vi "Apply Tombstone.vi"(5 "Time of Death (ToD)":timestamp, 7 "Grave Digger":string, 8 "Error In":errorcluster, 11 "Grave In":refnum<vi>) -> (0 "Error Out":errorcluster, 3 "Grave Out":refnum<vi>)   [LabVIEW 2017, in "Toolkit VIs.lvlib"]
doc: "Adds a tomestome to the grave. The grave is a Diagram Disable structure and the tomestone is its label as a bookmark with a \"RIP\" tag to indicate its a tomestone, the died date in YYYYMMDD format, and the name of the grave digger (programmer). \n\nBy default today's date is used as the died date and the application/system user name is used for the grave digger."
uses:
  Toolkit VIs.lvlib
  Public/Typedefs/Bookmark Tags.ctl
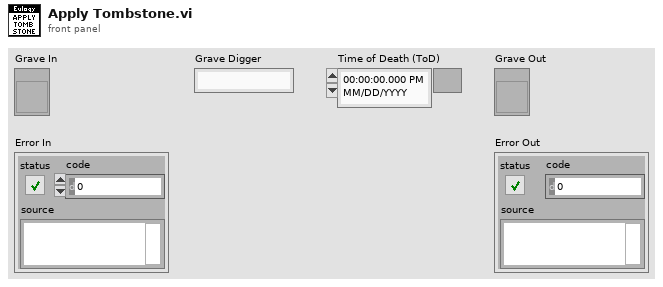
[diagram p1: front panel]
types:
  T1 = typedef "Toolkit VIs.lvlib/Bookmark Tags.ctl" = enum16{"RIP", "Zombie"}
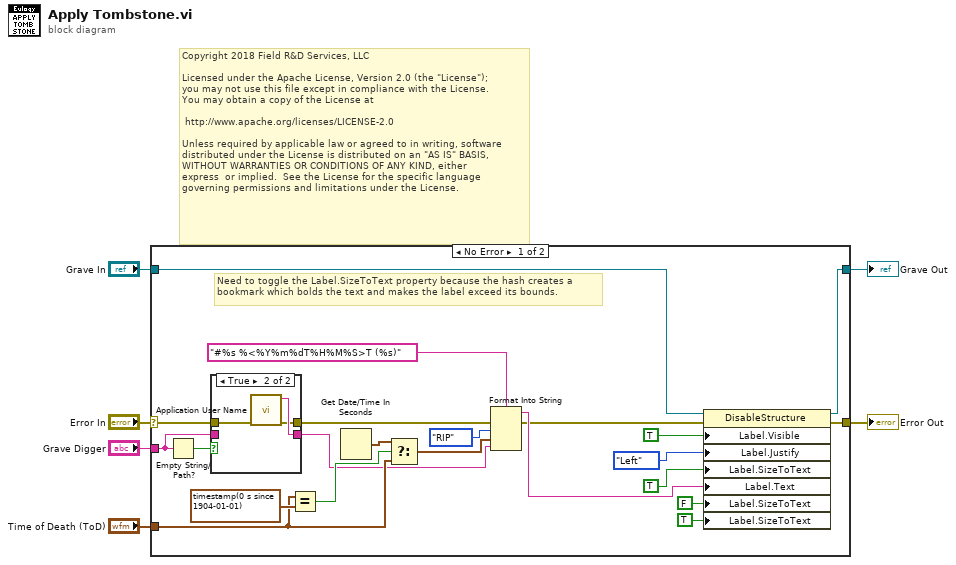
[diagram p0: block diagram]
diagram:
  # "Copyright 2018 Field R&D Services, LLC\n\nLicensed under the Apache License, Version 2.0 (the \"License\");\nyou may not use this file except in compliance with the License.\nYou may obtain a copy of the License at\n\n\thttp://www.apache.org/licenses/LICENSE-2.0\n\nUnless required by applicable law or agreed to in writing, software\ndistributed under the License is distributed on an \"AS IS\" BASIS,\nWITHOUT WARRANTIES OR CONDITIONS OF ANY KIND, either \nexpress  or implied.  See the License for the specific language \ngoverning permissions and limitations under the License."
  n1 = case shown="No Error" "Error In" {
    selector: "Error In" -> [w17 w34]
    tunnel: [w25 w35] -> w6
    tunnel: [w24 w34] -> w5
    tunnel: "Grave In" -> [w23 w35]
    tunnel: "Time of Death (ToD)" -> [w12 _]
    tunnel: "Grave Digger" -> [w10 _]
    frame No Error {
      # "Need to toggle the Label.SizeToText property because the hash creates a bookmark which bolds the text and makes the label exceed its bounds."
      n2 = Empty String/Path?(string/path=w10) -> (empty?=w11:bool)
      n3 = case shown="True" w11 {
        tunnel: w17 -> [w30 w33]
        tunnel: [w30 w31] -> w16
        tunnel: [w29 w32] -> w8
        tunnel: w10 -> [w29 _]
        frame False {
        }
        frame True {
          n4 = call "Application User Name.vi"("Error In"=w33) -> ("Error Out"=w31:errorcluster, "User Name"=w32:string)  [unwired: 9 in]
        }
      }
      n5 = Equal?(x=w12, y=timestamp(0 s since 1904-01-01)) -> (x = y?=w14:bool)
      n6 = Get Date/Time In Seconds() -> (seconds since 1Jan1904=w13:timestamp)
      n7 = Select(t=w13, s=w14, f=w12) -> (s? t:f=w9:timestamp)
      n8 = Format Into String(format string="#%s %<%Y%m%dT%H%M%S>T (%s)", error in=w16, Bookmark_Tags."RIP" ("Bookmark"), w9, w8) -> (resulting string=w28:string, error out=w27:errorcluster)  [unwired: 1 in]
      n9 = property class="DisableStructure"(reference=w23, error in=w27, "Label.Visible"=TRUE ("Label.Size to Text?"), "Label.Justify"=enum16{"Left", "Center", "Right"}."Left" ("Label.Justification"), "Label.SizeToText"=TRUE ("Label.Size to Text?"), "Label.Text"=w28, "Label.SizeToText"=FALSE ("Label.Size to Text?"), "Label.SizeToText"=TRUE ("Label.Size to Text?")) -> (reference out=w25:refnum<vi>, error out=w24:errorcluster)
    }
    frame Error {
    }
  }
  "Grave Out" <- w6
  "Error Out" <- w5
